vi "Day 12 Puzzle 1.vi"(11 "Path":path) -> ()   [LabVIEW 2021]
uses:
  <vilib>/Utility/file.llb/Read Delimited Spreadsheet (string).vi
panel:
  out "Array 6":cluster{"Array":i32[][]}[](array[cluster])
  out "size(s) 3":i32
  in  "stop":bool
  out "E Y pos":i32[](array[numeric])
  out "E X pos":i32[](array[numeric])
  out "Array 5":bool[](array[boolean])
  out "size(s) 2":i32
  out "Array 4":i32[](array[numeric])
  out "Array 3":i32[](array[numeric])
  out "Successful routes":cluster{i32[][]}[](array[cluster])
  out "Array 2":cluster{i32[][]}[](array[cluster])
  out "min value":i32
  out "size(s)":i32[](array[numeric])
  out "Array":string[][](array[string])
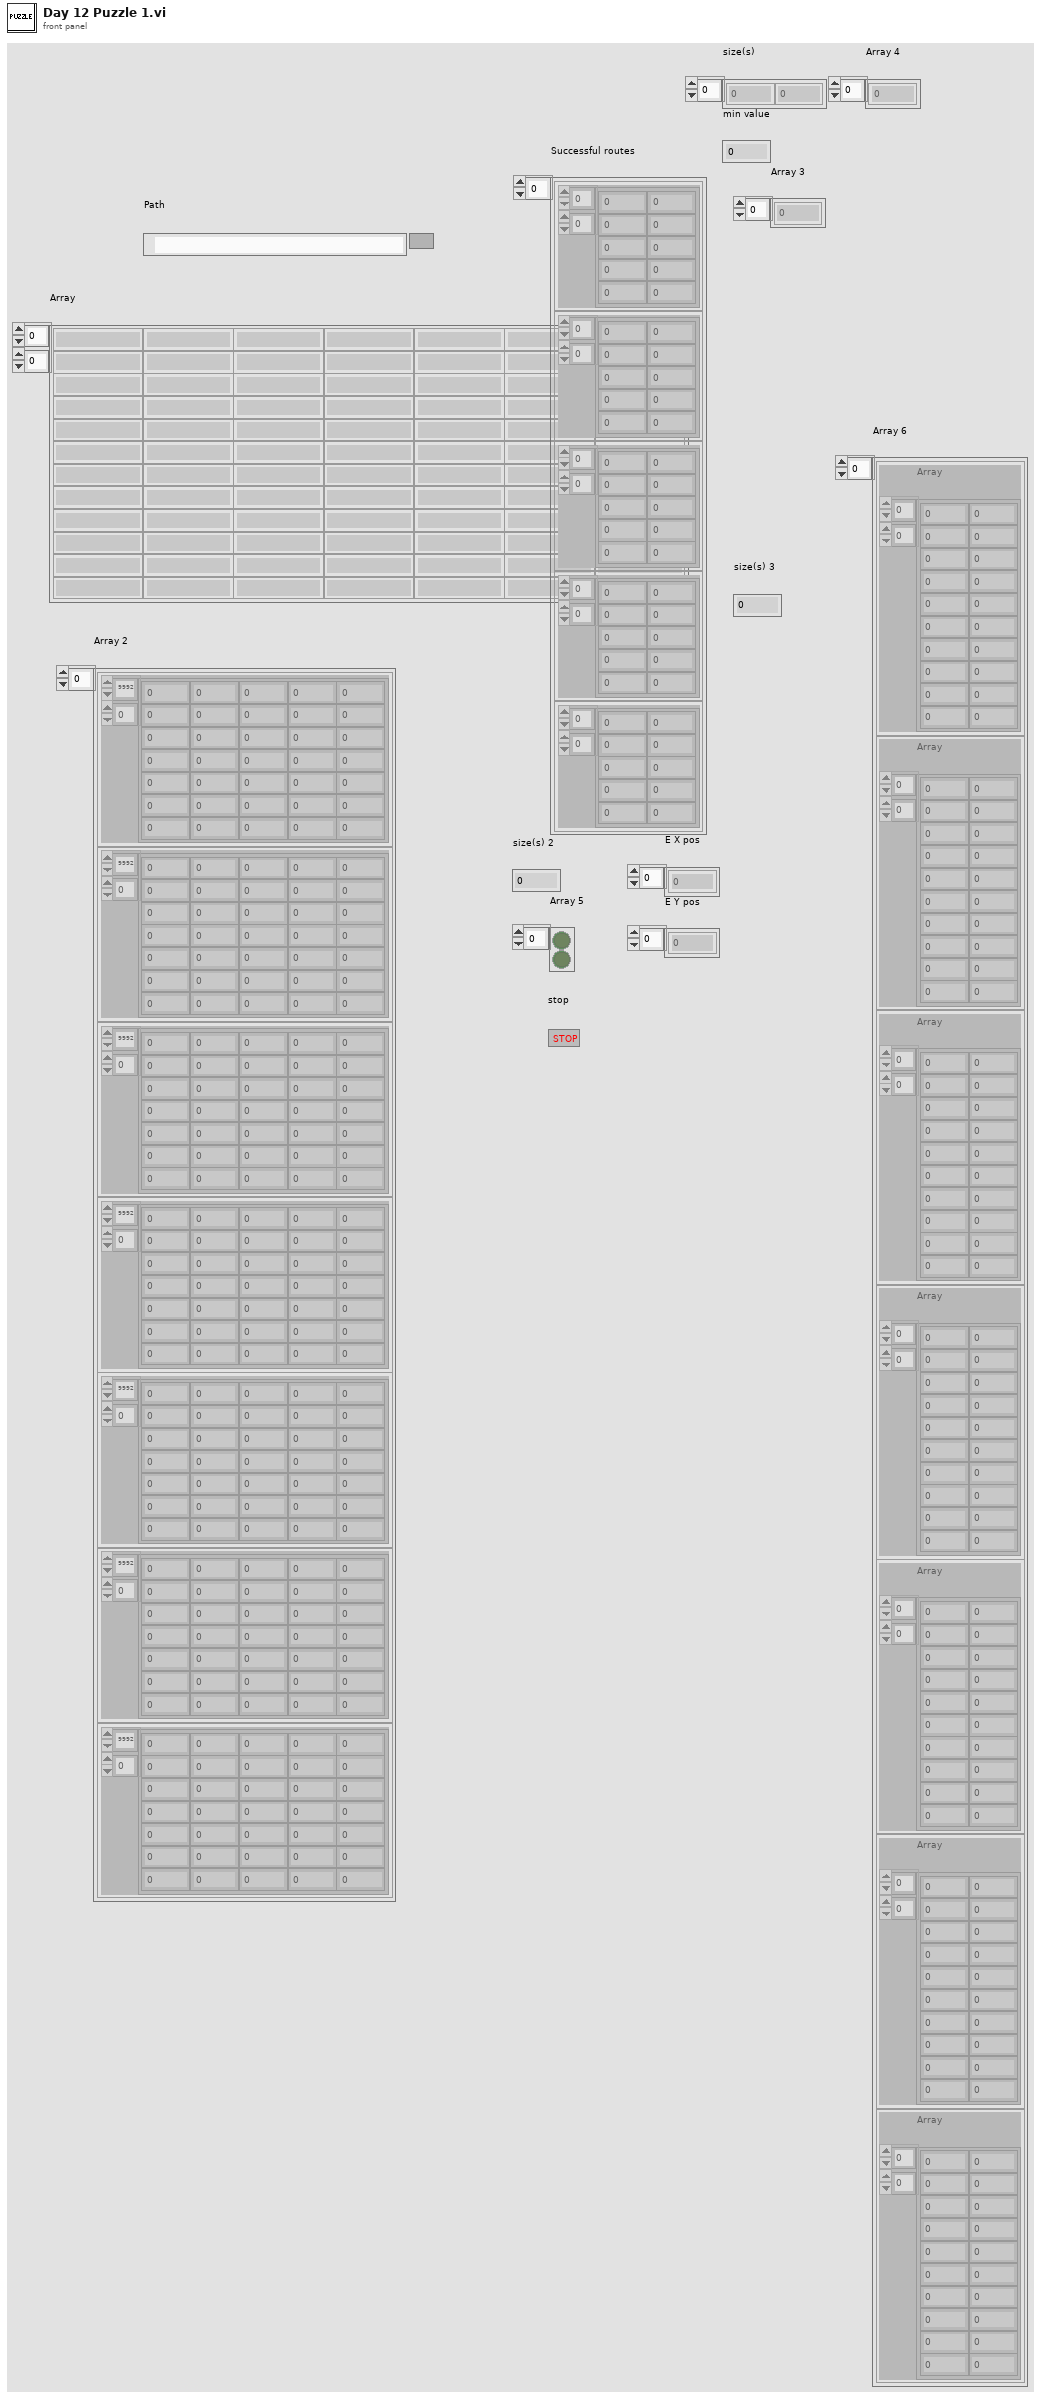
[diagram p1: front panel]
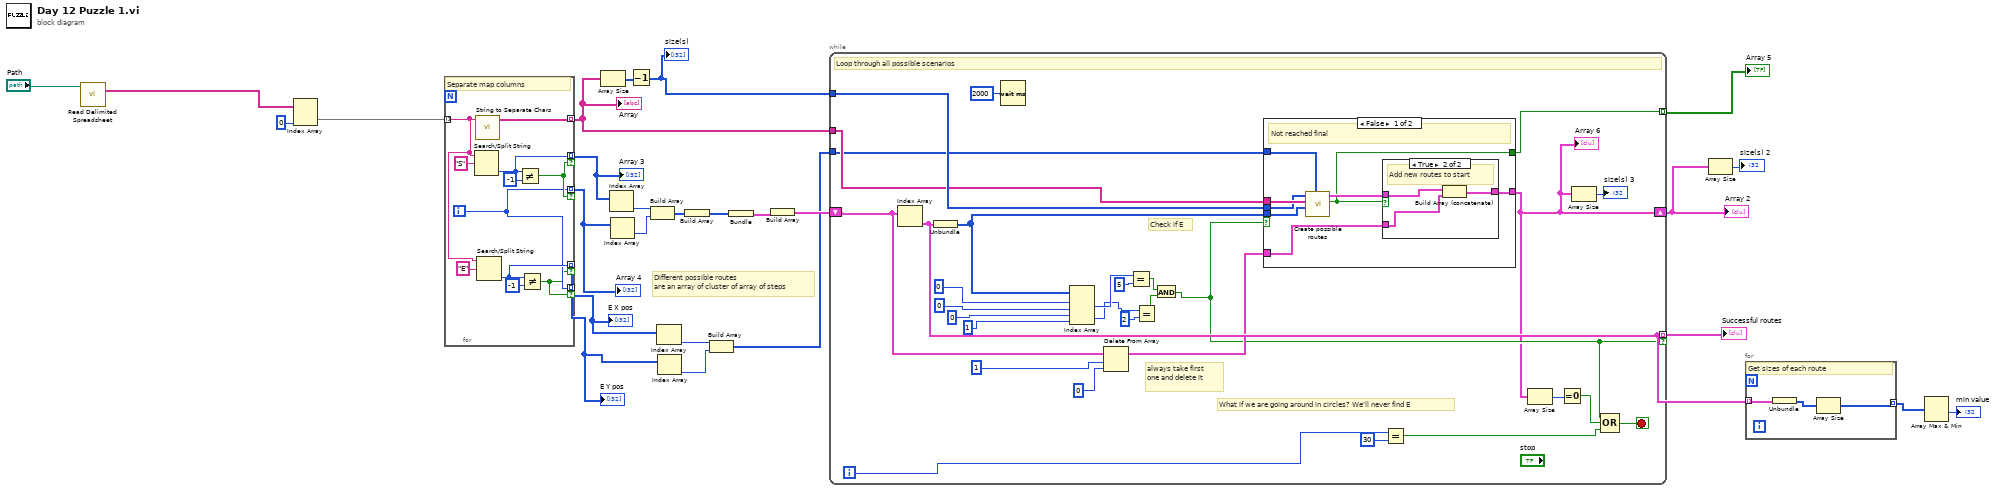
[diagram p0: block diagram]
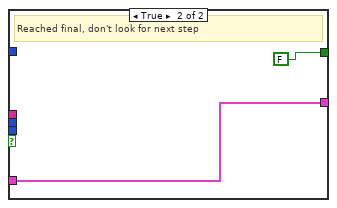
[diagram p3: hidden frame]
diagram:
  # "Different possible routes\nare an array of cluster of array of steps"
  n1 = call-poly <vilib>:"Read Delimited Spreadsheet.vi"("file path (dialog if empty)"="Path") -> ("all rows"=w25:string[][])  [unwired: 9 in, 5 out]
  n2 = Index Array(array=w25, index (col)=0 ("disabled index (col)")) -> (element=w23:string[])  [unwired: 1 in]
  n3 = for {
    tunnel: w23 -> [w30] mode=indexing
    tunnel: [w37] -> w16 mode=indexing
    tunnel: [w28] -> w9 mode=indexing if=w33
    tunnel: [w34] -> w22 mode=indexing if=w33
    tunnel: [w29] -> w5 mode=indexing if=w27
    tunnel: [w28] -> w4 mode=indexing if=w27
    i -> [w28]
    # "Separate map columns"
    n4 = Search/Split String(string=w30, search string/char (-)="S") -> (offset of match=w34:i32)  [unwired: 1 in, 2 out]
    n5 = call "String to Separate Chars.vi"("String"=w30) -> ("Array"=w37:string[])  [unwired: 10 in]
    n6 = Search/Split String(string=w30, search string/char (-)="E") -> (offset of match=w29:i32)  [unwired: 1 in, 2 out]
    n7 = Not Equal?(x=w34, y=-1) -> (x != y?=w33:bool)
    n8 = Not Equal?(x=w29, y=-1) -> (x != y?=w27:bool)
  }
  "Array" <- w16
  "Array 3" <- w22
  "Array 4" <- w9
  "E X pos" <- w5
  "E Y pos" <- w4
  n9 = Array Size(array=w16) -> (size(s)=w18:i32[])
  n10 = Index Array(array=w22) -> (element=w21:i32)  [unwired: 1 in]
  n11 = Index Array(array=w9) -> (element=w20:i32)  [unwired: 1 in]
  n12 = Decrement(x=w18) -> (x-1=w17:i32[])
  "size(s)" <- w17
  n13 = Build Array(w21, w20) -> (w11:i32[])
  n14 = Index Array(array=w5) -> (element=w3:i32)  [unwired: 1 in]
  n15 = Index Array(array=w4) -> (element=w2:i32)  [unwired: 1 in]
  n16 = Build Array(w11) -> (w10:i32[][])
  n17 = Build Array(w3, w2) -> (w1:i32[])
  n18 = Bundle(w10) -> (w15:cluster{i32[][]})  [unwired: 1 in]
  n19 = Build Array(w15) -> (w19:cluster{i32[][]}[])
  n20 = while {
    tunnel: w17 -> [w67]
    tunnel: w16 -> [w66]
    tunnel: [w65] -> w14 mode=indexing if=w45
    shift-right: [w43] -> w8
    shift-left: w19 -> [w62]
    tunnel: [w55] -> w6 mode=indexing
    tunnel: w1 -> [w54]
    i -> [w41]
    stop <- w44 stop-if-true
    # "What if we are going around in circles? We'll never find E"
    # "always take first one and delete it"
    # "Check if E"
    # "Loop through all possible scenarios"
    n21 = Index Array(array=w62) -> (element=w65:cluster{i32[][]})  [unwired: 1 in]
    n22 = Unbundle(w65) -> (w53:i32[][])
    n23 = Wait (ms)(milliseconds to wait=u32 2000) -> ()  [unwired: 1 out]
    n24 = Index Array(array=w53, index (row) #1=0 ("index (row)"), index (col) #1=0 ("disabled index (col)"), index (row) #2=0 ("index (row)"), index (col) #2=1 ("disabled index (col)")) -> (element #1=w52:i32, element #2=w49:i32)
    n25 = Delete From Array(array=w62, length=1, index=0) -> (array with subset deleted=w61:cluster{i32[][]}[])  [unwired: 1 out]
    n26 = Equal?(x=w52, y=5) -> (x = y?=w48:bool)
    n27 = Equal?(x=w49, y=2) -> (x = y?=w47:bool)
    n28 = And(x=w48, y=w47) -> (x .and. y?=w45:bool)
    n29 = case shown="False" w45 {
      tunnel: w67 -> [w71 _]
      tunnel: w66 -> [w75 _]
      tunnel: w53 -> [w70 _]
      tunnel: w61 -> [w73 w81]
      tunnel: [w72 w81] -> w43
      tunnel: [w69 FALSE] -> w55
      tunnel: w54 -> [w68 _]
      frame False {
        # "Not reached final"
        n30 = call "Create possible routes.vi"("Aim position"=w68, "Route"=w70, "Map"=w75, "Plot Sizes"=w71) -> ("Carry on route?"=w69:bool, "New routes"=w74:cluster{"Array":i32[][]}[])  [unwired: 6 in]
        n31 = case shown="True" w69 {
          tunnel: w74 -> [_ w78]
          tunnel: w73 -> [w76 w77]
          tunnel: [w76 w79] -> w72
          frame False {
            # "End route"
          }
          frame True {
            # "Add new routes to start"
            n32 = Build Array (concatenate)(w78, w77) -> (w79:cluster{"Array":i32[][]}[])
          }
        }
      }
      frame True {
        # "Reached final, don't look for next step"
      }
    }
    "Array 6" <- w43
    n33 = Equal?(x=w41, y=30) -> (x = y?=w39:bool)
    n34 = Array Size(array=w43) -> (size(s)=w60:i32)
    n35 = Equal To 0?(x=w60) -> (x = 0?=w46:bool)
    n36 = Array Size(array=w43) -> (size(s)=→"size(s) 3":i32)
    n37 = Compound Arithmetic op=OR(w45, w46, w39) -> (w44:bool)
  }
  "Array 2" <- w8
  "Successful routes" <- w14
  "Array 5" <- w6
  n38 = Array Size(array=w8) -> (size(s)=→"size(s) 2":i32)
  n39 = for {
    tunnel: w14 -> [w84] mode=indexing
    tunnel: [w82] -> w13 mode=indexing
    # "Get sizes of each route"
    n40 = Unbundle(w84) -> (w83:i32[][])
    n41 = Array Size(array=w83) -> (size(s)=w82:i32[])
  }
  n42 = Array Max & Min(array=w13) -> (min value=→"min value":i32)  [unwired: 3 out]
